vi "New.vi"(8 "Error In":errorcluster, 11 "Key":string) -> (0 "Error Out":errorcluster, 3 "Escaped Variable":refnum<class "EscapedVariable.lvclass">)   [LabVIEW 2017, in "Mustache.lvlib" / "Tokens.lvlib" / "EscapedVariable.lvclass"]
uses:
  EscapedVariable.lvclass
  EscapedVariable.lvclass/EscapedVariable.ctl
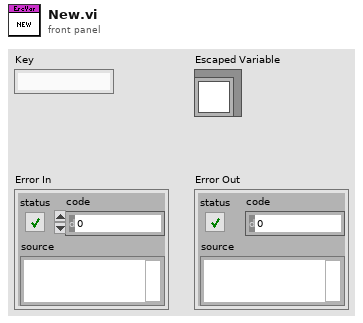
[diagram p1: front panel]
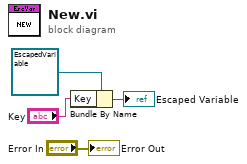
[diagram p0: block diagram]
diagram:
  n1 = Bundle By Name(cluster=refnum<class "EscapedVariable.lvclass"> refnum ("Mustache.lvlib:Tokens.lvlib:Tag.lvclass"), "Key"="Key") -> (→"Escaped Variable":refnum<class "EscapedVariable.lvclass">)
  "Error Out" <- "Error In"
